vi "GetSpectrometerArrays.vi"(8 "error in (no error)":errorcluster, 11 "Instruments in":refnum<class "Instruments.lvclass">) -> (0 "error out":errorcluster, 1 "Spectrum":dbl[](array[numeric]), 2 "Wavelength":dbl[](array[numeric]), 3 "Instruments out":refnum<class "Instruments.lvclass">)   [LabVIEW 2012, in "Instruments.lvclass"]
uses:
  Instruments.lvclass
  Instruments.lvclass/Instruments.ctl
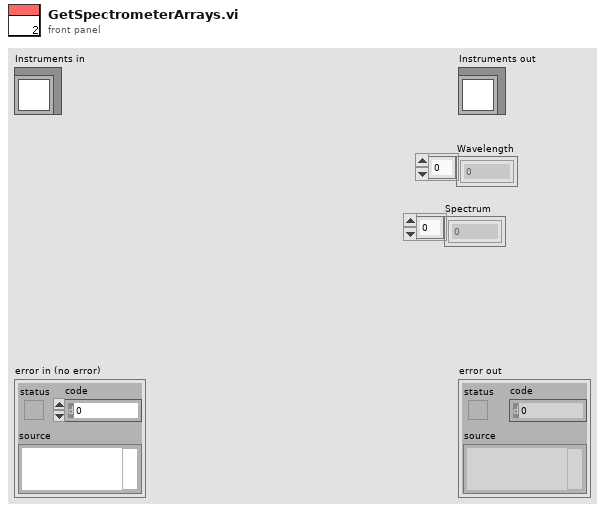
[diagram p1: front panel]
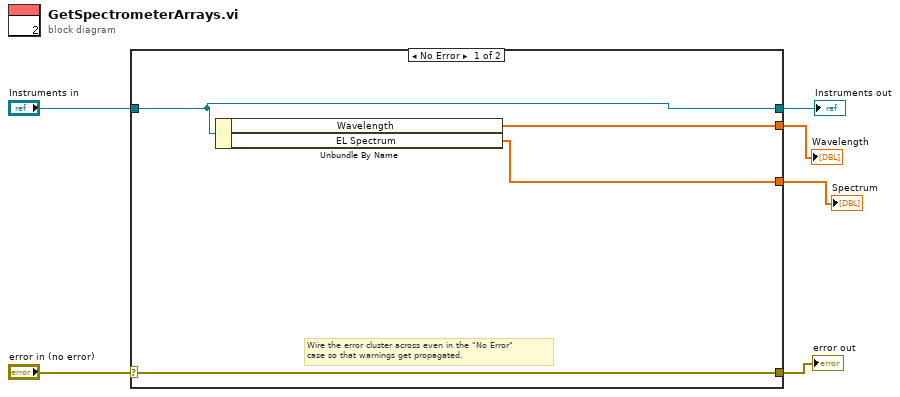
[diagram p0: block diagram]
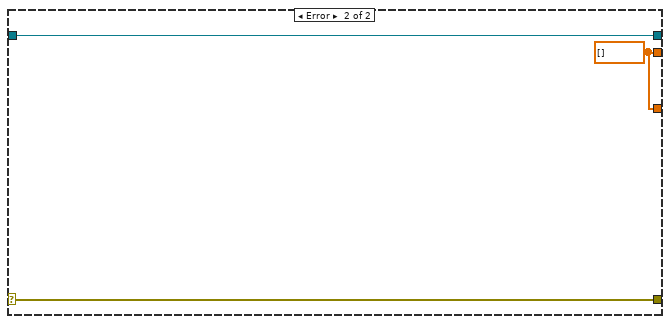
[diagram p2: hidden frame]
diagram:
  n1 = case shown="No Error" "error in (no error)" {
    selector: "error in (no error)" -> [w10 w13]
    tunnel: [w10 w13] -> w5
    tunnel: [w9 w12] -> w3
    tunnel: "Instruments in" -> [w9 w12]
    tunnel: [w8 w11] -> w2
    tunnel: [w7 w11] -> w1
    frame No Error {
      # "Wire the error cluster across even in the \"No Error\"\ncase so that warnings get propagated."
      n2 = Unbundle By Name(w9) -> ("Wavelength"=w8:dbl[], "EL Spectrum"=w7:dbl[])
    }
    frame Error {
      w11 = dbl[] [] ("Wavelength")
    }
  }
  "error out" <- w5
  "Instruments out" <- w3
  "Wavelength" <- w2
  "Spectrum" <- w1
